vi "EX6.vi"() -> ()   [LabVIEW 2018]
panel:
  out "seuille = 10":bool
  in  "OK Button":bool
  in  "Operation":T1(ring)
  out "Result":dbl
  in  "B":dbl
  in  "A":dbl
  out "date string":string
  out "time string":string
  # "EX6 - TP0"
  # "Mekni Marwen 2ème Année Génie Electrique"
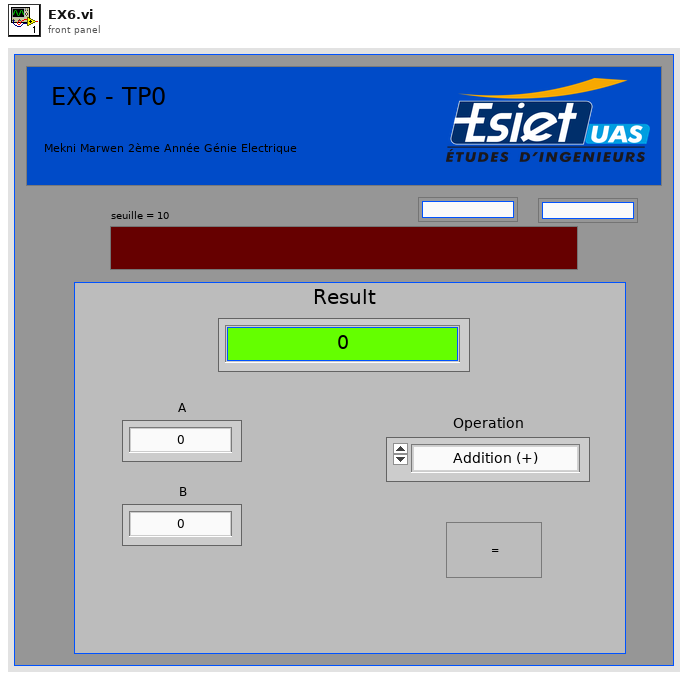
[diagram p1: front panel]
types:
  T1 = enum16{"Addition (+)", "Subtraction (-)", "Multiplication (×)", "Division (÷)"}
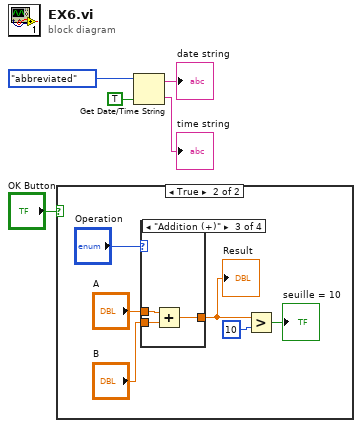
[diagram p0: block diagram]
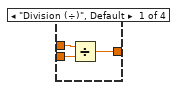
[diagram p3: hidden frame]
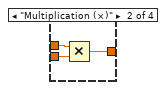
[diagram p4: hidden frame]
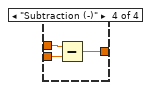
[diagram p5: hidden frame]
diagram:
  n1 = case shown="True" "OK Button" {
    frame False {
    }
    frame True {
      n2 = case shown="\"Addition (+)\"" "Operation" {
        tunnel: "A" -> [w14 w17 w19 w22]
        tunnel: "B" -> [w13 w16 w18 w21]
        tunnel: [w12 w15 w20 w23] -> w7
        frame "Division (÷)", Default {
          n3 = Divide(x=w14, y=w13) -> (x/y=w12:dbl)
        }
        frame "Multiplication (×)" {
          n4 = Multiply(x=w17, y=w16) -> (x*y=w15:dbl)
        }
        frame "Addition (+)" {
          n5 = Add(x=w19, y=w18) -> (x+y=w20:dbl)
        }
        frame "Subtraction (-)" {
          n6 = Subtract(x=w22, y=w21) -> (x-y=w23:dbl)
        }
      }
      "Result" <- w7
      n7 = Greater?(x=w7, y=10) -> (0:→"seuille = 10":bool)
    }
  }
  n8 = Get Date/Time String(date format (0)=enum16{"short", "long", "abbreviated"}."abbreviated", want seconds? (F)=TRUE) -> (date string=→"date string":string, time string=→"time string":string)  [unwired: 1 in]
